vi "ClusterToJSON.vi"(11 "cluster":T1={"SI camera info"={"Observer Name"="", "object name"="", "File name base"="", "Camera Color"="Red", "Exp type tab"="", "Number of Exp"=1, "Exp time"=0, "CCD Readout Speed"=5, "CCD ROI Mode"=10, "Hg(Ar)"=FALSE, "Cu"=FALSE, "Ne"=FALSE, "Bulb"=FALSE, "Ar"=FALSE, "Quartz"=FALSE, "Quartz Percent"=0, "Fe"=FALSE, "Notes"="", "Target Number"="", "DomePercent"=0, "Dome"=FALSE, "Start"=0.0, "Delta"=0.0, "Steps"=0.0}, "Configuration"={"Primary Filter"="<NO FILTER>", "Secondary Filter"="<NO FILTER>", "Slit Mask"="<NO MASK>", "Grating"="<NO GRATING>", "CS Target"=0.0, "GS Target"=0.0, "Coll Focus"=1000, "Camera Focus"=0, "Name"="", "User"="", "Date"="", "Comment"="", "use Flexure Comp?"=FALSE, "Select Mode:"=0}} {"Configuration"."Select Mode:" items=["Custom", "Imaging", "300 All", "600 UV", "600 Blue", "600 Mid", "600 Red", "1200 m0", "1200 m1", "1200 m2", "1200 m3", "1200 m4", "1200 m5", "1200 m6", "1200 m7", "1200 RESOLVE", "400 m1", "400 m2", "930 m1", "930 m2", "930 m3", "930 m4", "930 m5", "930 m6", "400WD", "930TP", "400Fermi", "400Padgett", "400Lewis", "400Crotts", "600BLee", "600RLee", "400WW"]; "SI camera info"."DomePercent" min=0 step=1; "SI camera info"."Quartz Percent" min=0 step=1; "SI camera info"."CCD Readout Speed" items=["750 kHz, ATTN 0", "750 kHz, ATTN 2", "344 kHz, ATTN 0", "344 kHz, ATTN 3", "100 kHz, ATTN 2", "100 kHz, ATTN 3"]; "SI camera info"."CCD ROI Mode" items=["Imaging, 1x1  "=0, "Imaging, 2x2"=1, "Imaging, 3x3"=2, "Spectroscopic, 1x1"=3, "Spectroscopic, 2x2"=4, "Spectroscopic, 3x3"=5, "MOS, 1x1"=11, "MOS, 2x2"=12, "MOS, 3x3"=13, "Slicer"=6, "Spectroscopic, ZZ Ceti"=14, "Slit Imaging/Alignment"=7, "MOS Imaging/Alignment"=10, "Set user-defined ROI..."=21, "Custom Mode"=9]; "SI camera info"."Number of Exp" min=0 step=1; "SI camera info"."Exp time" min=0 step=1}) -> (3 "out":string)   [LabVIEW 2015]
panel:
  in  "Path to Configuration File":path
  # "Or"
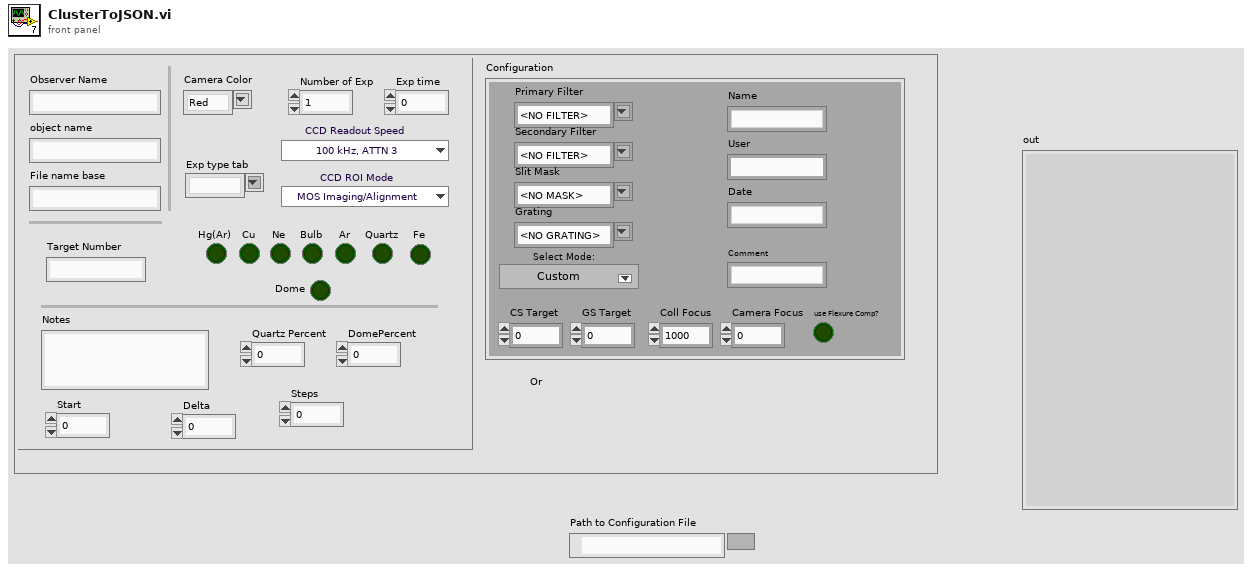
[diagram p1: front panel]
types:
  T1 = cluster{"SI camera info":cluster{"Observer Name":string, "object name":string, "File name base":string, "Camera Color":string, "Exp type tab":string, "Number of Exp":i32, "Exp time":i32, "CCD Readout Speed":u8, "CCD ROI Mode":u16, "Hg(Ar)":bool, "Cu":bool, "Ne":bool, "Bulb":bool, "Ar":bool, "Quartz":bool, "Quartz Percent":i32, "Fe":bool, "Notes":string, "Target Number":string, "DomePercent":i32, "Dome":bool, "Start":dbl, "Delta":dbl, "Steps":dbl}, "Configuration":cluster{"Primary Filter":string, "Secondary Filter":string, "Slit Mask":string, "Grating":string, "CS Target":dbl, "GS Target":dbl, "Coll Focus":i32, "Camera Focus":i32, "Name":string, "User":string, "Date":string, "Comment":string, "use Flexure Comp?":bool, "Select Mode:":u16}}
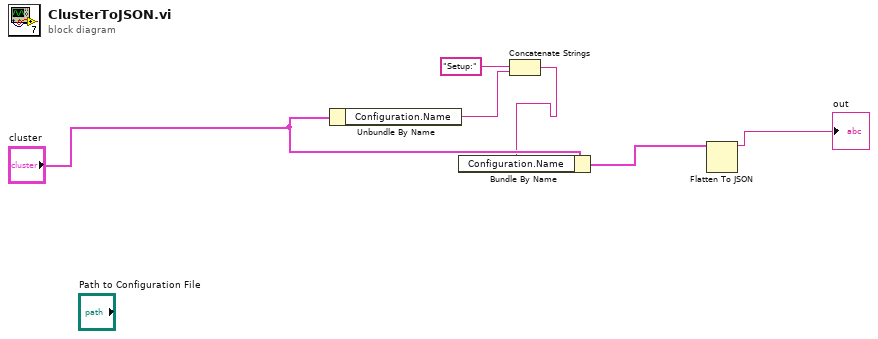
[diagram p0: block diagram]
diagram:
  n1 = Unbundle By Name("cluster") -> ("Configuration.Name"=w5:string)
  n2 = Concatenate Strings("Setup:", w5) -> (w3:string)
  n3 = Bundle By Name(cluster="cluster", "Configuration.Name"=w3) -> (w2:T1)
  n4 = Flatten To JSON(anything=w2) -> (JSON string=→"out":string)  [unwired: 2 in, 1 out]
